vi "Test Region.vi"(11 "Test Case In":refnum<class "Test.Camera.lvclass">) -> (0 "error out":errorcluster, 3 "Test Case Out":refnum<class "Test.Camera.lvclass">)   [LabVIEW 2020, in "Test.Camera.lvclass"]
uses:
  Test.Camera.lvclass
  C:/Program Files (x86)/National Instruments/LabVIEW 2020/vi.lib/Astemes/LUnit/Test Case.lvclass
  g_industrial_cam/Camera/Camera.lvclass/Camera.ctl
  <vilib>/Astemes/LUnit/Test Case.lvclass/Test Case.ctl
  g_industrial_cam/Buffer/Image Size.ctl
  g_industrial_cam/Camera/Image Offset.ctl
  c3e2611f-c54f-4219-a549-b8da21c7f085.vi
  0aa1576c-e916-4ad0-9a97-64bd3e4eb69b.vi
  g_industrial_cam/Camera/GetSetRegion.vi
  <vilib>/Astemes/LUnit/Core/LUnit Test Case/Private/Append Pass Result.vi
  <vilib>/Astemes/LUnit/Core/LUnit Test Case/Private/Append Fail Result.vi
  0aa1576c-e916-4ad0-9a97-64bd3e4eb69b.vi/9c5d11cd-9439-4240-a1ee-d9baace9c924.vi
  <vilib>/Astemes/LUnit/Core/LUnit Test Case/Private/Run In UI.vi
  <vilib>/Utility/error.llb/Clear Errors.vi
  g_industrial_cam/Camera/Check Not Disconnected.vi
  <vilib>/Utility/error.llb/Error Cluster From Error Code.vi
  Test.Camera.lvclass/Test.Camera.ctl
  <vilib>/Astemes/LUnit/Test Case.lvclass
  g_industrial_cam/Camera/Camera.lvclass
  g_industrial_cam/Buffer/Buffer.lvclass
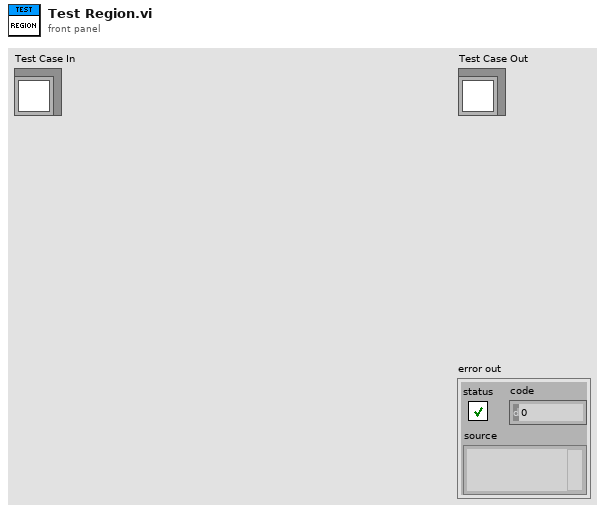
[diagram p1: front panel]
types:
  T1 = typedef "Buffer.lvclass/Image Size.ctl" = cluster{"Width":u16, "Height":u16}
  T2 = typedef "Camera.lvclass/Image Offset.ctl" = cluster{"x":i32, "y":i32}
  T3 = cluster{"Y Offset Increment":i32, "Y Offset Min":i32, "Y Offset Max":i32, "X Offset Increment":i32, "X Offset Min":i32, "X Offset Max":i32, "Offset Avaliable":bool, "Height Increment":i32, "Height Min":i32, "Height Max":i32, "Width Increment":i32, "Width Min":i32, "Width Max":i32, "Sensor Size":T1, "Region Offset":T2, "Region Size":T1}
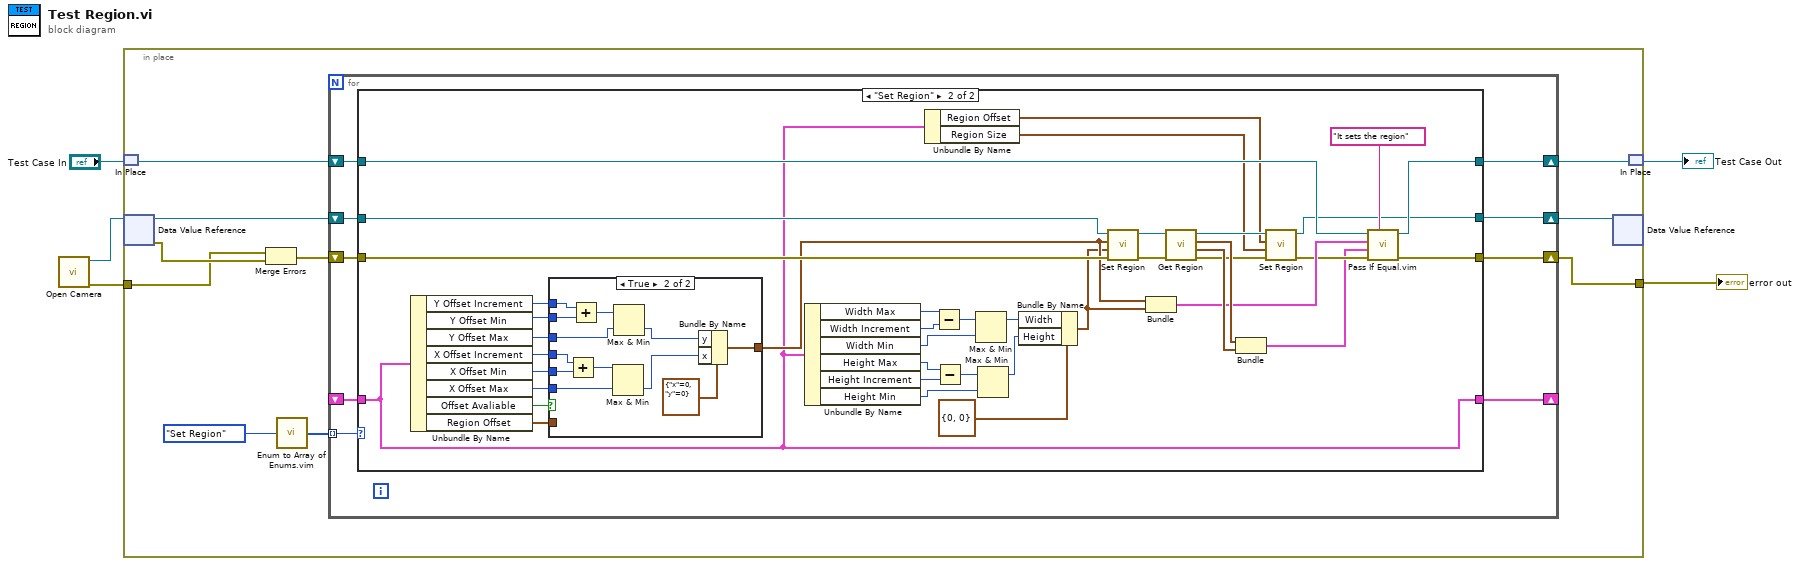
[diagram p0: block diagram]
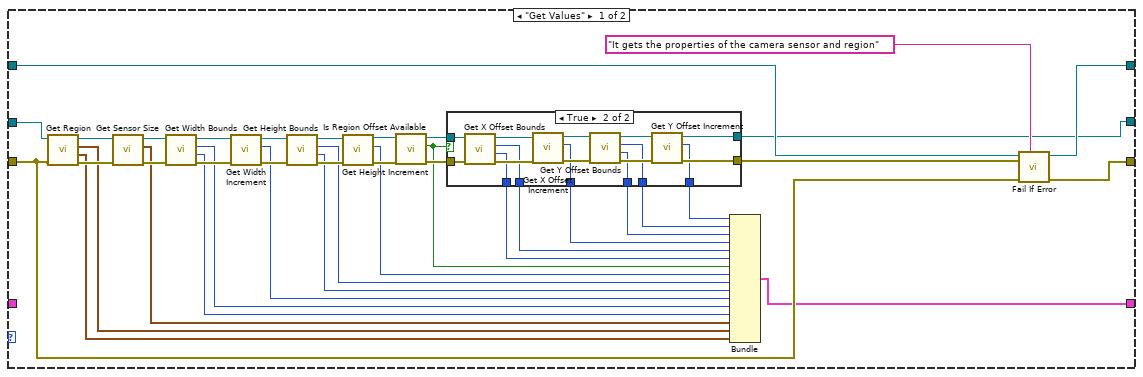
[diagram p2: hidden frame]
diagram:
  n1 = call "Open Camera.vi"() -> ("error out"=w5:errorcluster, "Camera"=w4:refnum<data-value>)  [unwired: 10 in]
  n2 = in-place {
    in-place-border: w5 -> [w8]
    in-place-border: [w7] -> w2
    n3 = in-place-match #1("Test Case In") -> (w10:refnum<class "Test.Camera.lvclass">)
    n4 = in-place-dvr #2(w4) -> (w14:refnum<class "Camera.lvclass">, w15:errorcluster)
    n5 = Merge Errors(w8, w15) -> (w13:errorcluster)
    n6 = call "Enum to Array of Enums.vim"("enum"=enum16{"Get Values", "Set Region"}."Set Region") -> ("array of enums"=w11:enum16{"Get Values", "Set Region"}[])
    n7 = for {
      tunnel: w11 -> [w22] mode=indexing
      shift-right: [w21] -> w9
      shift-left: w14 -> [w24]
      shift-right: [w20] -> _
      shift-left: _ -> [w19]
      shift-right: [w17] -> w6
      shift-left: w10 -> [w18]
      shift-right: [w16] -> w7
      shift-left: w13 -> [w23]
      n8 = case shown="\"Set Region\"" w22 {
        tunnel: w24 -> [w57 w98]
        tunnel: w23 -> [w58 w97]
        tunnel: [w25 w82] -> w21
        tunnel: [w26 w87] -> w20
        tunnel: w19 -> [_ w87]
        tunnel: w18 -> [w62 w99]
        tunnel: [w61 w121] -> w17
        tunnel: [w59 w120] -> w16
        frame "Get Values" {
          n9 = call "Get Region.vi"("error in (no error)"=w58, "Camera in"=w57) -> ("error out"=w63:errorcluster, "Region Size"=w56:T1, "Region Offset"=w55:T2, "Camera"=w54:refnum<class "Camera.lvclass">)  [unwired: 6 in]
          n10 = call "Get Sensor Size.vi"("error in (no error)"=w63, "Camera in"=w54) -> ("error out"=w51:errorcluster, "Sensor Size"=w45:T1, "Camera"=w53:refnum<class "Camera.lvclass">)  [unwired: 7 in]
          n11 = call "Get Width Bounds.vi"("error in (no error)"=w51, "Camera in"=w53) -> ("error out"=w50:errorcluster, "Width Max"=w44:i32, "Width Min"=w43:i32, "Camera"=w52:refnum<class "Camera.lvclass">)  [unwired: 6 in]
          n12 = call "Get Width Increment.vi"("error in (no error)"=w50, "Camera in"=w52) -> ("error out"=w49:errorcluster, "Width Increment"=w42:i32, "Camera"=w48:refnum<class "Camera.lvclass">)  [unwired: 7 in]
          n13 = call "Get Height Bounds.vi"("error in (no error)"=w49, "Camera in"=w48) -> ("error out"=w47:errorcluster, "Height Max"=w41:i32, "Height Min"=w40:i32, "Camera"=w46:refnum<class "Camera.lvclass">)  [unwired: 6 in]
          n14 = call "Get Height Increment.vi"("error in (no error)"=w47, "Camera in"=w46) -> ("error out"=w39:errorcluster, "Height Increment"=w37:i32, "Camera"=w38:refnum<class "Camera.lvclass">)  [unwired: 7 in]
          n15 = call "Is Region Offset Available.vi"("error in (no error)"=w39, "Camera in"=w38) -> ("error out"=w36:errorcluster, "Offset Avaliable"=w27:bool, "Camera"=w35:refnum<class "Camera.lvclass">)  [unwired: 7 in]
          n16 = case shown="True" w27 {
            tunnel: w36 -> [w65 w81]
            tunnel: w35 -> [w64 w80]
            tunnel: [_ w73] -> w34
            tunnel: [_ w72] -> w33
            tunnel: [_ w71] -> w32
            tunnel: [_ w70] -> w31
            tunnel: [_ w69] -> w30
            tunnel: [w65 w68] -> w29
            tunnel: [_ w67] -> w28
            tunnel: [w64 w66] -> w25
            frame False {
            }
            frame True {
              n17 = call "Get X Offset Bounds.vi"("error in (no error)"=w81, "Camera in"=w80) -> ("error out"=w79:errorcluster, "X Offset Max"=w73:i32, "X Offset Min"=w72:i32, "Camera"=w76:refnum<class "Camera.lvclass">)  [unwired: 6 in]
              n18 = call "Get X Offset Increment.vi"("error in (no error)"=w79, "Camera in"=w76) -> ("error out"=w78:errorcluster, "X Offset Increment"=w71:i32, "Camera"=w75:refnum<class "Camera.lvclass">)  [unwired: 7 in]
              n19 = call "Get Y Offset Bounds.vi"("error in (no error)"=w78, "Camera in"=w75) -> ("error out"=w77:errorcluster, "Y Offset Max"=w70:i32, "Y Offset Min"=w69:i32, "Camera"=w74:refnum<class "Camera.lvclass">)  [unwired: 6 in]
              n20 = call "Get Y Offset Increment.vi"("error in (no error)"=w77, "Camera in"=w74) -> ("error out"=w68:errorcluster, "Y Offset Increment"=w67:i32, "Camera"=w66:refnum<class "Camera.lvclass">)  [unwired: 7 in]
            }
          }
          n21 = Bundle("Y Offset Increment"=w28, "Y Offset Min"=w30, "Y Offset Max"=w31, "X Offset Increment"=w32, "X Offset Min"=w33, "X Offset Max"=w34, "Offset Avaliable"=w27, "Height Increment"=w37, "Height Min"=w40, "Height Max"=w41, "Width Increment"=w42, "Width Min"=w43, "Width Max"=w44, "Sensor Size"=w45, "Region Offset"=w55, "Region Size"=w56) -> (w26:T3)  [unwired: 1 in]
          n22 = call <vilib>:"Fail If Error.vi"("Description"="It gets the properties of the camera sensor and region", "error in (no error)"=w58, "Assert error"=w29, "LUnit Test Case In"=w62) -> ("error out"=w59:errorcluster, "LUnit Test Case Out"=w61:refnum<class "Test.Camera.lvclass">)  [unwired: 6 in]
        }
        frame "Set Region" {
          n23 = Unbundle By Name(w87) -> ("Y Offset Increment"=w116:i32, "Y Offset Min"=w117:i32, "Y Offset Max"=w113:i32, "X Offset Increment"=w114:i32, "X Offset Min"=w115:i32, "X Offset Max"=w112:i32, "Offset Avaliable"=w118:bool, "Region Offset"=w111:T2)
          n24 = case shown="True" w118 {
            tunnel: [w122 w123] -> w94
            tunnel: w117 -> [_ w134]
            tunnel: w116 -> [_ w133]
            tunnel: w115 -> [_ w132]
            tunnel: w114 -> [_ w131]
            tunnel: w113 -> [_ w129]
            tunnel: w112 -> [_ w127]
            tunnel: w111 -> [w122 _]
            frame False {
            }
            frame True {
              n25 = Add(x=w131, y=w132) -> (x+y=w128:i32)
              n26 = Add(x=w133, y=w134) -> (x+y=w130:i32)
              n27 = Max & Min(x=w128, y=w127) -> (min(x,y)=w126:i32)  [unwired: 1 out]
              n28 = Max & Min(x=w130, y=w129) -> (min(x,y)=w125:i32)  [unwired: 1 out]
              n29 = Bundle By Name(cluster=T2 {"x"=0, "y"=0} ("Image Offset"), "y"=w125, "x"=w126) -> (w123:T2)
            }
          }
          n30 = Unbundle By Name(w87) -> ("Width Max"=w110:i32, "Width Increment"=w109:i32, "Width Min"=w105:i32, "Height Max"=w108:i32, "Height Increment"=w107:i32, "Height Min"=w103:i32)
          n31 = Unbundle By Name(w87) -> ("Region Offset"=w86:T2, "Region Size"=w85:T1)
          n32 = Subtract(x=w110, y=w109) -> (x-y=w106:i32)
          n33 = Subtract(x=w108, y=w107) -> (x-y=w104:i32)
          n34 = Max & Min(x=w106, y=w105) -> (max(x,y)=w101:i32)  [unwired: 1 out]
          n35 = Max & Min(x=w104, y=w103) -> (max(x,y)=w100:i32)  [unwired: 1 out]
          n36 = Bundle By Name(cluster=T1 {"Width"=0, "Height"=0} ("Image Size"), "Width"=w101, "Height"=w100) -> (w93:T1)
          n37 = call "Set Region.vi"("error in (no error)"=w97, "Image Size"=w93, "Image Offset"=w94, "Camera in"=w98) -> ("error out"=w96:errorcluster, "Camera"=w95:refnum<class "Camera.lvclass">)  [unwired: 6 in]
          n38 = Bundle("Image Offset"=w94, "Image Size"=w93) -> (w90:cluster{"Image Offset":T2, "Image Size":T1})  [unwired: 1 in]
          n39 = call "Get Region.vi"("error in (no error)"=w96, "Camera in"=w95) -> ("error out"=w89:errorcluster, "Region Size"=w91:T1, "Region Offset"=w92:T2, "Camera"=w88:refnum<class "Camera.lvclass">)  [unwired: 6 in]
          n40 = Bundle("Region Offset"=w92, "Region Size"=w91) -> (w83:cluster{"Region Offset":T2, "Region Size":T1})  [unwired: 1 in]
          n41 = call "Set Region.vi"("error in (no error)"=w89, "Image Size"=w85, "Image Offset"=w86, "Camera in"=w88) -> ("error out"=w84:errorcluster, "Camera"=w82:refnum<class "Camera.lvclass">)  [unwired: 6 in]
          n42 = call "Pass If Equal.vim"("Description"="It sets the region", "error in (no error)"=w84, "Actual"=w83, "Expected"=w90, "LUnit Test Case In"=w99) -> ("error out"=w120:errorcluster, "LUnit Test Case Out"=w121:refnum<class "Test.Camera.lvclass">)  [unwired: 5 in]
        }
      }
    }
    n43 = in-place-dvr #2(w9) -> ()  [unwired: 2 out]
    n44 = in-place-match #1(w6) -> (→"Test Case Out":refnum<class "Test.Camera.lvclass">)
  }
  "error out" <- w2
